vi "libssh2_session_flag.vi"(8 "error in (no error)":errorcluster, 9 "value (0 = disabled)":i32, 10 "flag":T1, 11 "session":T2) -> (0 "error out":errorcluster)   [LabVIEW 2013, in "libssh2.lvlib"]
doc: "Set the value of a session flag."
uses:
  libssh2.lvlib
  Session Refnum.ctl
  libssh2_flag.ctl
  Not A Session.vi
  <vilib>/Utility/error.llb/Error Cluster From Error Code.vi
  Global Settings.vi
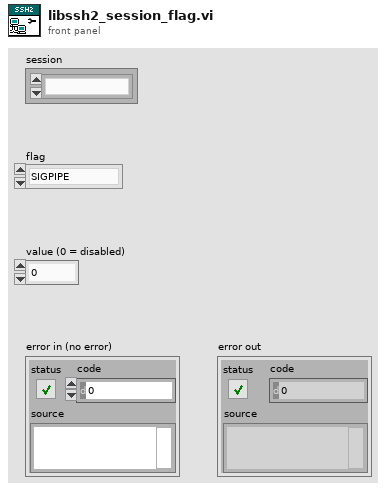
[diagram p1: front panel]
types:
  T1 = typedef "libssh2.lvlib/libssh2_flag.ctl" = enum16{"SIGPIPE", "COMPRESS", "QUOTE_PATHS"}
  T2 = typedef "libssh2.lvlib/Session Refnum.ctl" = refnum<k1>
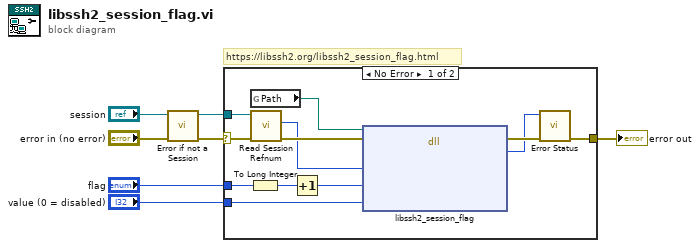
[diagram p0: block diagram]
diagram:
  # "https://libssh2.org/libssh2_session_flag.html"
  n1 = call "Error if not a Session.vi"("error in (no error)"="error in (no error)", "session"="session") -> ("error out"=w5:errorcluster, "session out"=w3:T2)  [unwired: 8 in]
  n2 = case shown="No Error" w5 {
    selector: w5 -> [w18 w20]
    tunnel: [w13 w20] -> w7
    tunnel: w3 -> [w17 _]
    tunnel: "flag" -> [w11 _]
    tunnel: "value (0 = disabled)" -> [w8 _]
    frame No Error {
      n3 = To Long Integer(number=w11) -> (32bit integer=w10:i32)
      n4 = global read "Global Settings.vi" "Path"() -> (w14:path)
      n5 = call "Read Session Refnum.vi"("error in (no error)"=w18, "session"=w17) -> ("error out"=w16:errorcluster, "LIBSSH2_SESSION*"=w15:u64)  [unwired: 5 in, 3 out]
      n6 = Increment(x=w10) -> (x+1=w9:i32)
      n7 = dll-call lib="?" fn="libssh2_session_flag"(path in=w14, error in=w16, "session"=w15, "flag"=w9, "value"=w8) -> (error out=w19:errorcluster, "return value"=w12:i32)  [unwired: 4 in, 1 out]
      n8 = call "Error Status.vi"("error in (no error)"=w19, "return value"=w12) -> ("error out"=w13:errorcluster)  [unwired: 8 in, 1 out]
    }
    frame Error {
    }
  }
  "error out" <- w7
